vi "R45crio2_fpga.vi"() -> ()   [LabVIEW 2016]
uses:
  <vilib>/LabVIEW Targets/FPGA/cRIO/shared/nicrio_ModuleControls/nicrio_cRIO-9871_BaudRateEnum.ctl
  <vilib>/LabVIEW Targets/FPGA/cRIO/shared/nicrio_ModuleControls/nicrio_cRIO-9871_DataBitsEnum.ctl
  <vilib>/LabVIEW Targets/FPGA/cRIO/shared/nicrio_ModuleControls/nicrio_cRIO-9871_StopBitsEnum.ctl
  <vilib>/LabVIEW Targets/FPGA/cRIO/shared/nicrio_ModuleControls/nicrio_cRIO-9871_ParityEnum.ctl
  <vilib>/Platform/TimedLoop/XDataNode/timing_clust.ctl
  <vilib>/Platform/TimedLoop/XDataNode/nitl_modes.ctl
  <vilib>/Platform/TimedLoop/XDataNode/wakeup.ctl
  <vilib>/rvi/FXPMathLib/basic elements/FxpIntAccumulator/subVIs/nifxpmath_IntAccumulator_SimConfig.ctl
  <vilib>/rvi/Emulation/niFpgaGetClockAttributes.vi
  <vilib>/rvi/Emulation/niFpgaSctlEmulationGetInTimedLoop.vi
  <vilib>/rvi/Emulation/niFpgaEmulationReportErrorSimple.vi
  <vilib>/rvi/eio/common/nirviEmuTemplateMethod_errors.vi
  <vilib>/rvi/Emulation/niFpgaCriticalErrorInLSC.vi
  <vilib>/rvi/Analysis/common/codeGenErrors/XNode/niFpgaXNodeCodeGenErrorHandle.vi
  <vilib>/rvi/FXPMathLib/basic elements/FxpIntAccumulator/simVIs/DllFxpIntAccumulator_sub.vi
  <vilib>/rvi/eio/common/nirviEmuTemplatePropertySet_noerrors.vi
  <vilib>/eio/EIONode/EIONode.xnode
  <vilib>/eio/EIOMethodNode/EIOMethodNode.xnode
  <vilib>/rvi/Analysis/measure/dc-rms/XNode/niFpgaDC-RMS.xnode
  <vilib>/Platform/TimedLoop/XDataNode/XDataNode.xnode
  <vilib>/rvi/FXPMathLib/basic elements/FxpIntAccumulator/XNode/nifxpmath_IntAccumulator.xnode
  <vilib>/rvi/FXPMathLib/FxpMul/XNode/nifxpmath_Multiplier.xnode
  <vilib>/eio/EIOPropertyNode/EIOPropertyNode.xnode
  <vilib>/Platform/TimedLoop/XDataNode/XDNodeRunTimeDep.lvlib
  <vilib>/rvi/FXPMathLib/sim/FxpSim.dll
  <vilib>/rvi/eio/common/nirviEmuTemplatePropertyGet_errors.vi
  <vilib>/rvi/eio/common/nirviEmuTemplatePropertyGet_noerrors.vi
  <vilib>/rvi/eio/common/nirviEmuTemplatePropertySet_errors.vi
panel:
  out "ig":bool
  out "cg gauge":bool
  in  "turbo valve R45 ExB":bool
  in  "beamline valve R45 detector":bool
  in  "turbo valve r45 det turbo":bool
  in  "turbo valve r45 waist":bool
  out "Data":u8
  out "Timed Out":bool
  out "gfm read":u8[](array[numeric])
  in  "gfm set field array":u8[](array[numeric])=[0, 0, 0, 0, 0, 0, 0, 0, 0, 0]
  out "Reset 2":bool
  in  "Reset":bool
  in  "exb ps set array 2":u8[](array[numeric])=[0, 0, 0, 0, 0, 0, 0, 0, 0, 0]
  out "r45 #4 Ion gauge 2":u8[](array[numeric])
  out "r45 #4 Convectron 2":u8[](array[numeric])
  out "r45 #4 Convectron 1":u8[](array[numeric])
  out "r45 #4 Ion gauge 1":u8[](array[numeric])
  out "r45 #3 Ion gauge 2":u8[](array[numeric])
  out "r45 #3 Convectron 2":u8[](array[numeric])
  out "r45 #3 Convectron 1":u8[](array[numeric])
  out "r45 #3 Ion gauge 1":u8[](array[numeric])
  out "r45 #2 Ion gauge 2":u8[](array[numeric])
  out "r45 #2 Convectron 2":u8[](array[numeric])
  out "r45 #2 Convectron 1":u8[](array[numeric])
  out "r45 #2 Ion gauge 1":u8[](array[numeric])
  in  "exb ps set array":u8[](array[numeric])=[0, 0, 0, 0, 0, 0, 0, 0, 0, 0]
  out "DIO OUTPUT":bool[](array[boolean])
  in  "R45 det  faraday cup":bool
  in  "R45 det Aperture":bool
  out "Analog input":fxp<+/-,26,5>[](array[numeric]) format="%.23g"
  in  "Analog Output":fxp<+/-,26,5>[](array[numeric])=[0.0, 0.0, 0.0, 0.0, 0.0, 0.0, 0.0, 0.0] format="%.23g"
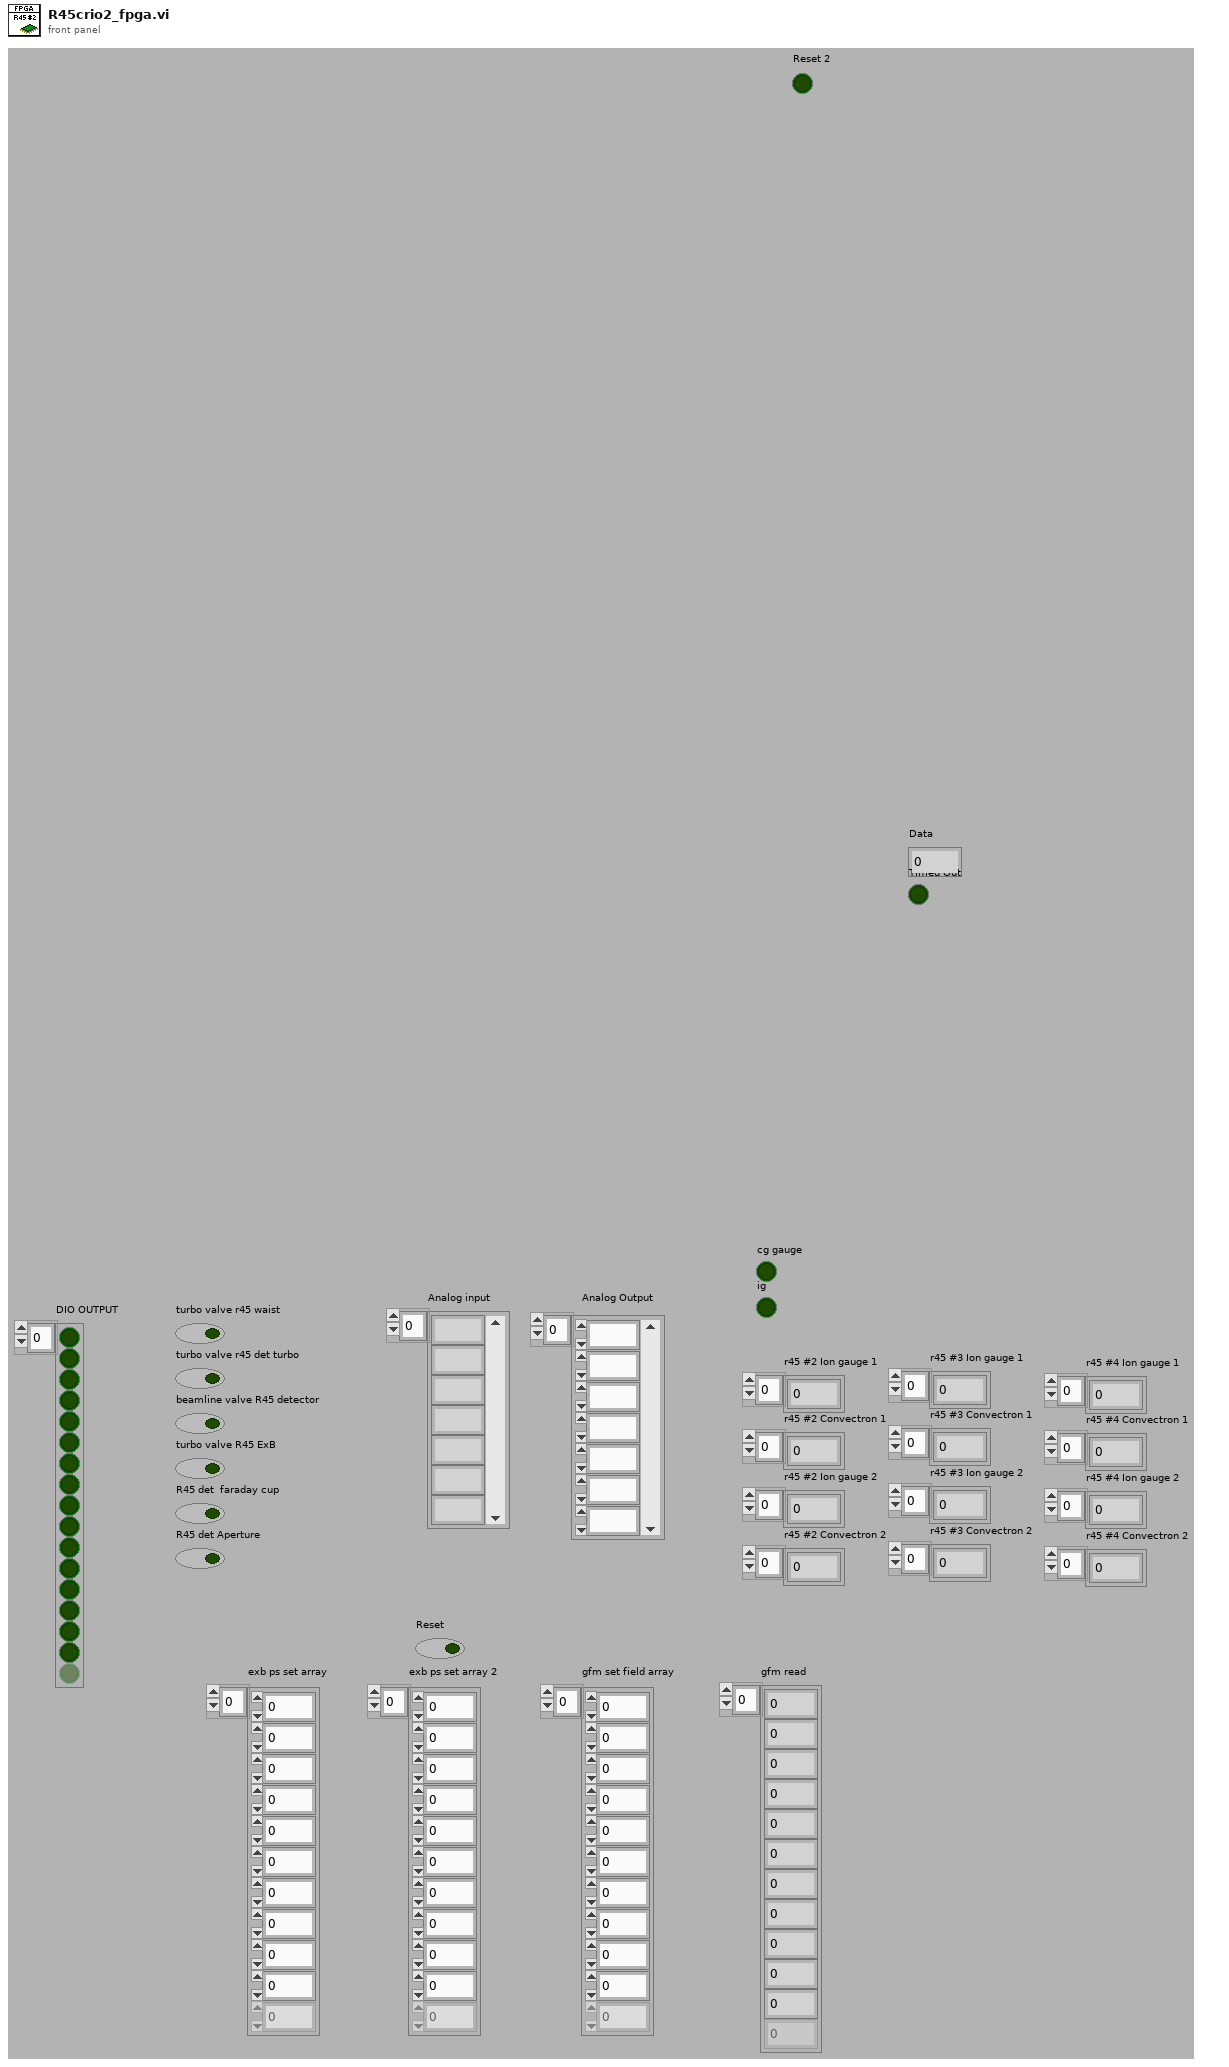
[diagram p1: front panel]
types:
  T1 = typedef "nicrio_cRIO-9871_ParityEnum.ctl" = enum8{"None", "Odd", "Even", "Mark", "Space"}
  T2 = typedef "nicrio_cRIO-9871_StopBitsEnum.ctl" = enum8{"1", "1.5", "2"}
  T3 = typedef "nicrio_cRIO-9871_BaudRateEnum.ctl" = enum16{"75 bps", "110 bps", "134 bps", "150 bps", "300 bps", "600 bps", "1200 bps", "1800 bps", "2400 bps", "4800 bps", "7200 bps", "9600 bps", "14.4 kbps", "19.2 kbps", "28.8 kbps", "38.4 kbps", "57.6 kbps", "115.2 kbps", "230.4 kbps", "460.8 kbps", "921.6 kbps"}
  T4 = typedef "nicrio_cRIO-9871_DataBitsEnum.ctl" = enum8{"5", "6", "7", "8"}
  T5 = typedef "XDNodeRunTimeDep.lvlib/timing_clust.ctl" = cluster{"Expected End [f-1]":u64, "Actual End [f-1]":u64, "Finished Late? [f-1]":bool, "Expected End [i-1]":u64, "Actual End [i-1]":u64, "Finished Late? [i-1]":bool, "Expected Start [i]":u64, "Actual Start [i]":u64, "Expected Start [f]":u64, "Actual Start [f]":u64, "Source Name":string, "Structure Name":string, "Period":i64, "Deadline":i64, "Offset":i64, "Start":i64, "Priority":i32, "Timeout":i32, "Mode":T6, "Wakeup Reason":T7, "Error":errorcluster, "Source Type":string, "Secondary Source Type":string, "Global End Time":u64, "Global Start Time":u64, "Frame Duration":u64, "Iteration Duration":u64, "Assigned CPU":i32, "I/O Scan Engine Mode":u32}
  T6 = typedef "XDNodeRunTimeDep.lvlib/nitl_modes.ctl" = enum32{"No Change", "Process missed periods, maintain original phase", "Discard missed periods, maintain original phase", "Process missed periods, ignore original phase", "Discard missed periods, ignore original phase"}
  T7 = typedef "XDNodeRunTimeDep.lvlib/wakeup.ctl" = enum32{"Normal", "Aborted", "Asynchronous wakeup", "Timing source error", "Timed loop error", "Timeout"}
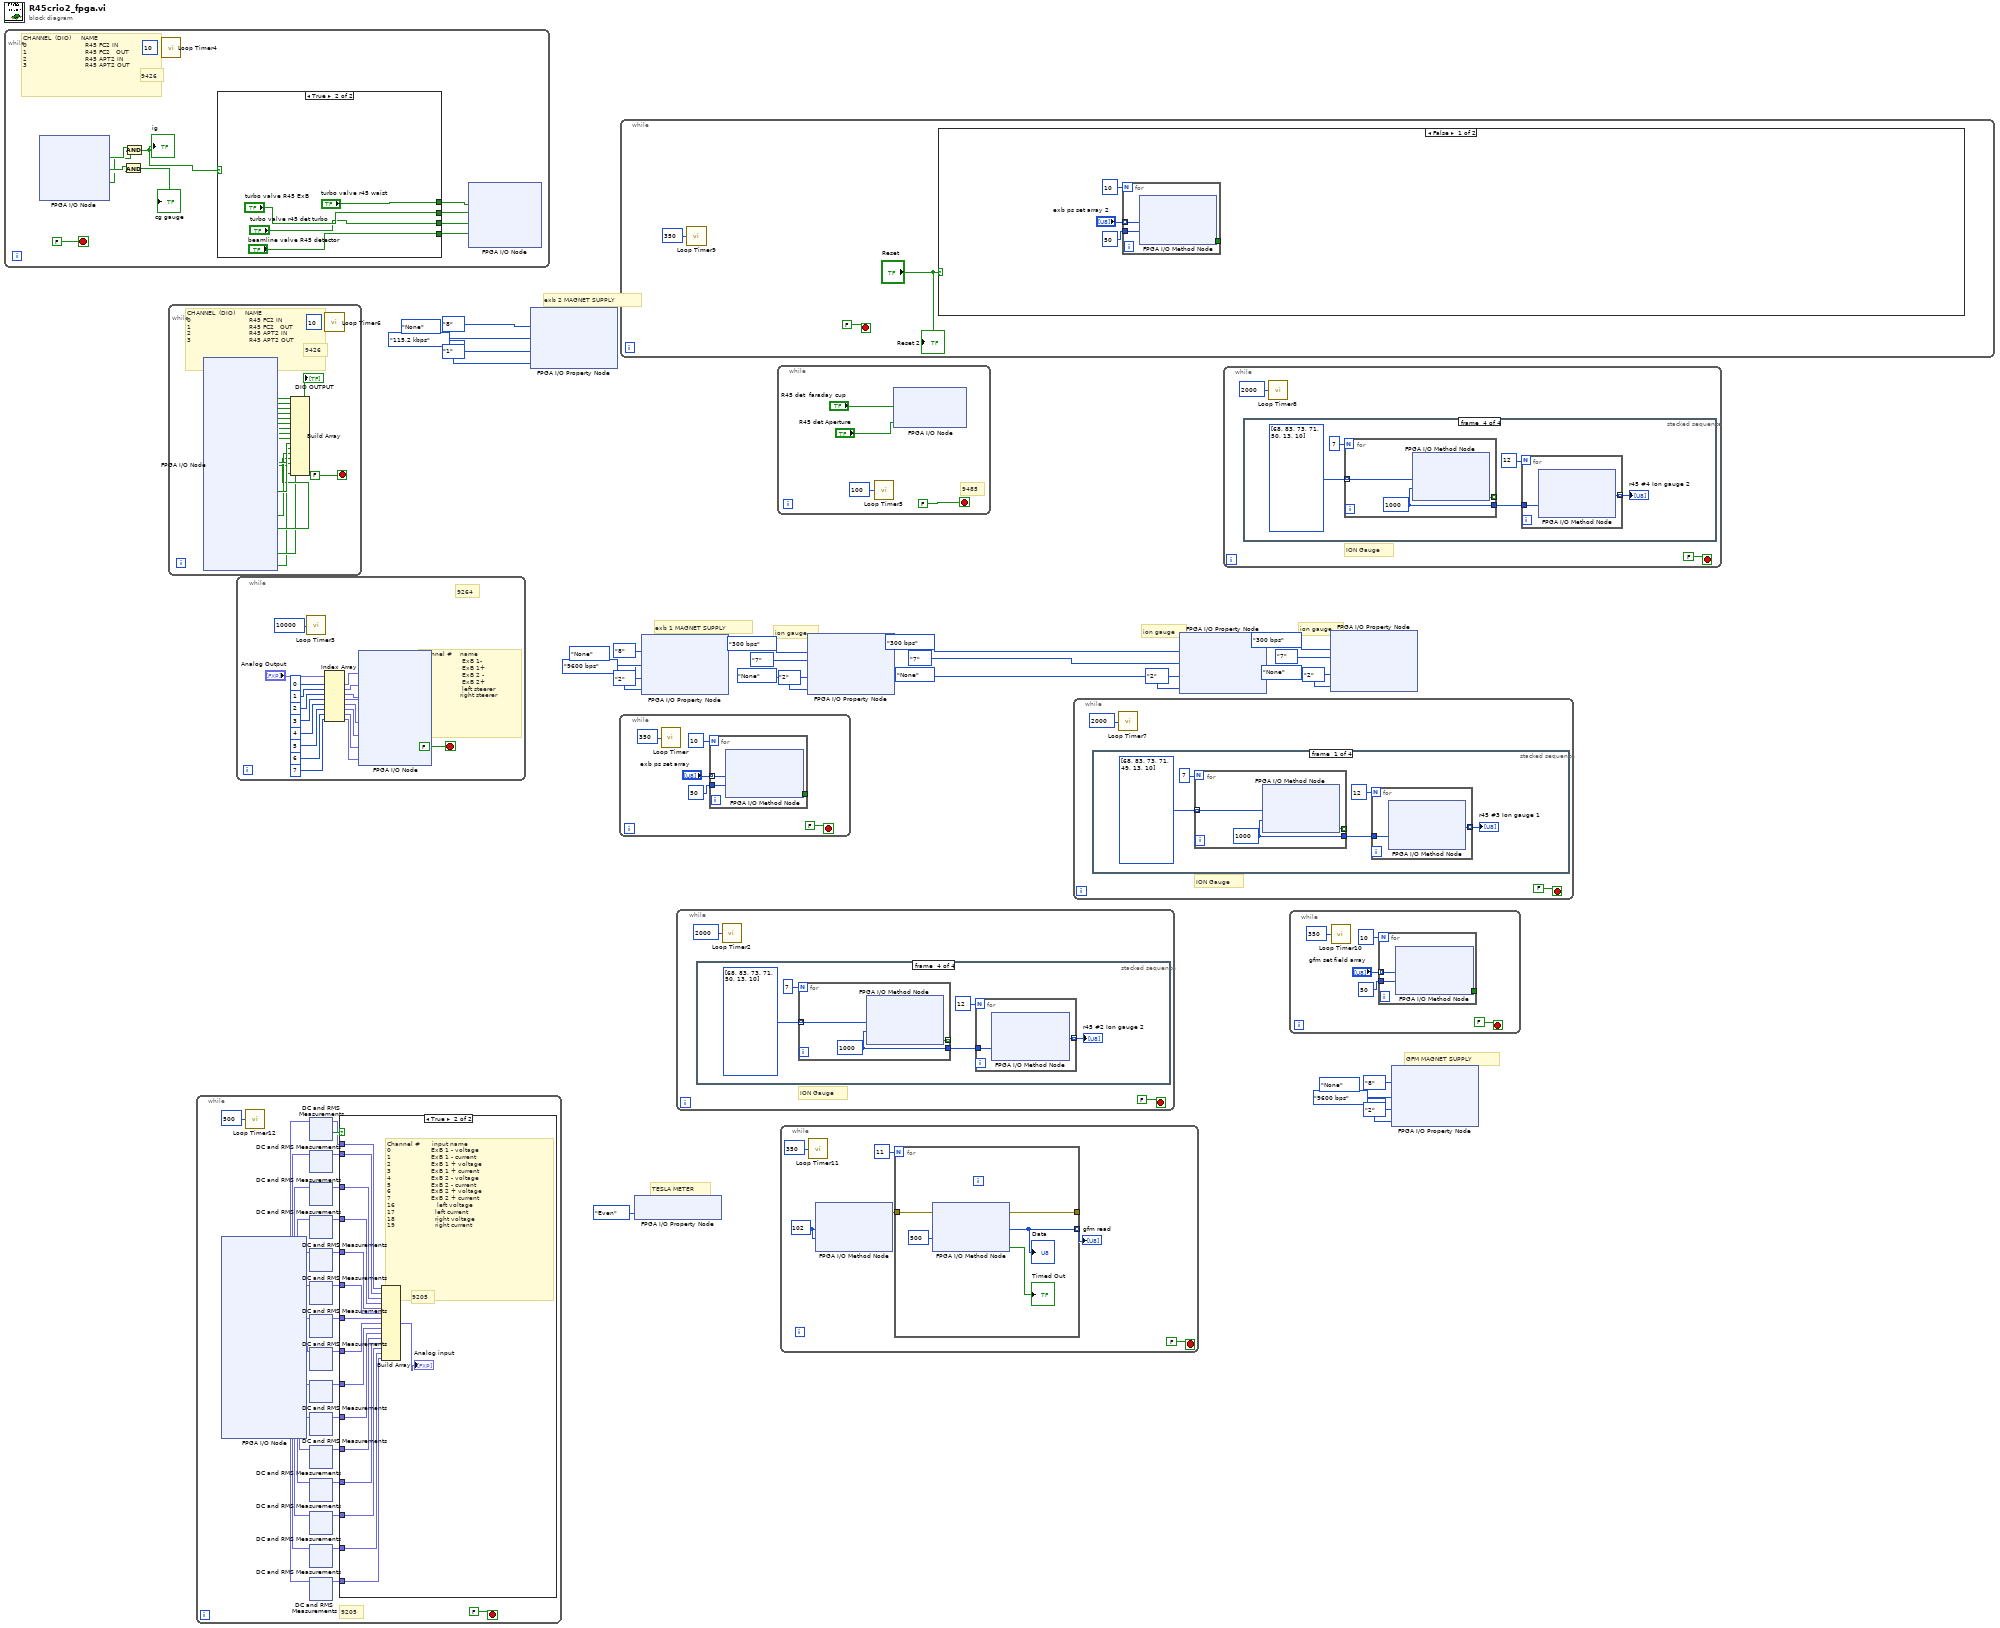
[diagram p0: block diagram]
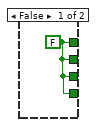
[diagram p2: hidden frame]
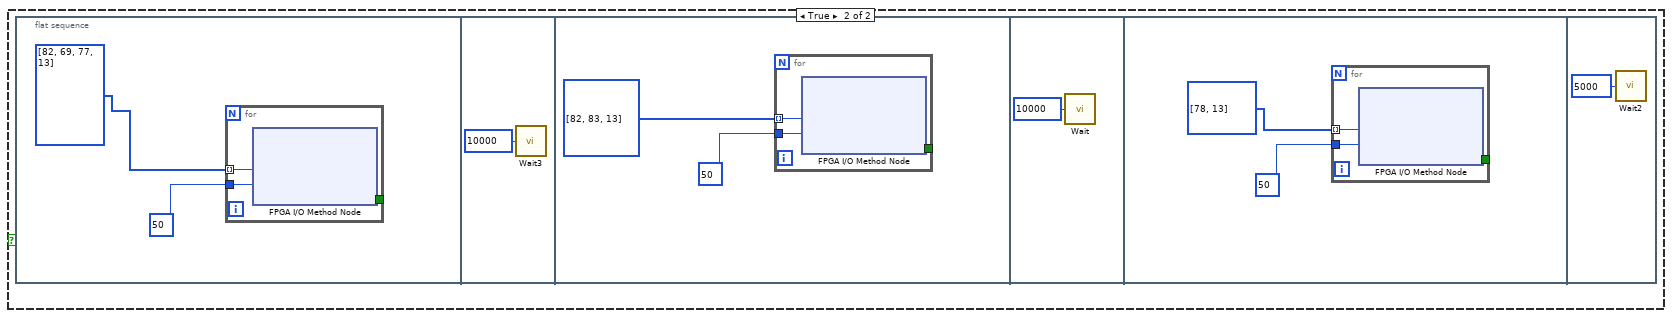
[diagram p4: hidden frame]
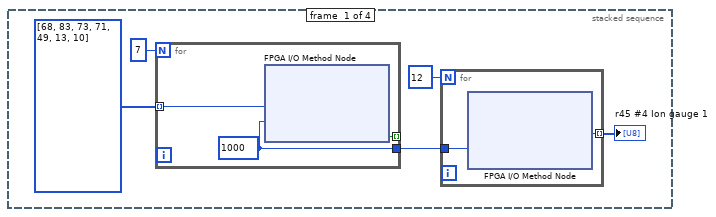
[diagram p5: hidden frame]
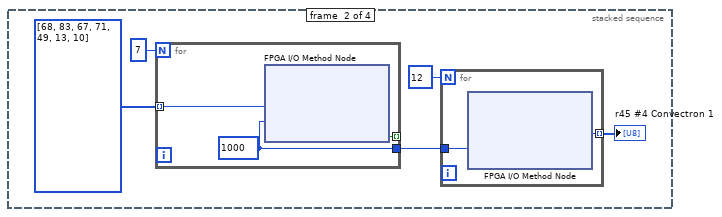
[diagram p6: hidden frame]
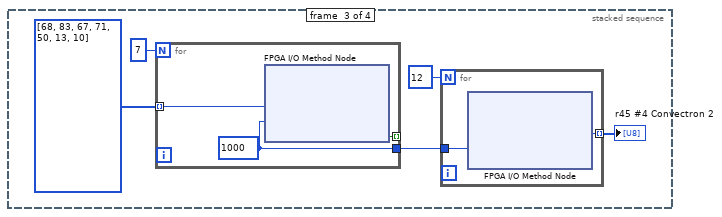
[diagram p7: hidden frame]
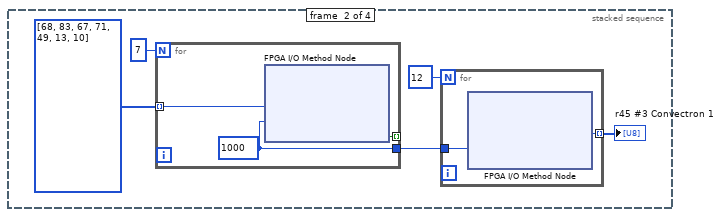
[diagram p8: hidden frame]
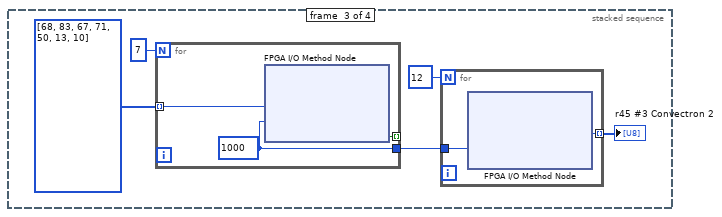
[diagram p9: hidden frame]
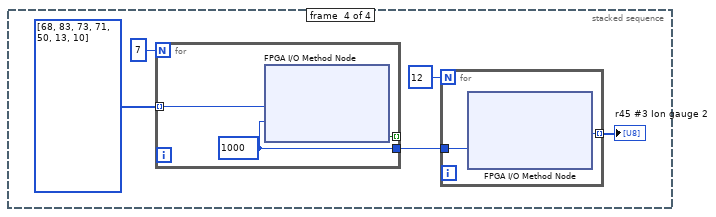
[diagram p10: hidden frame]
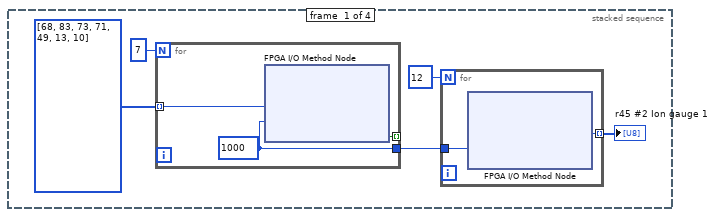
[diagram p11: hidden frame]
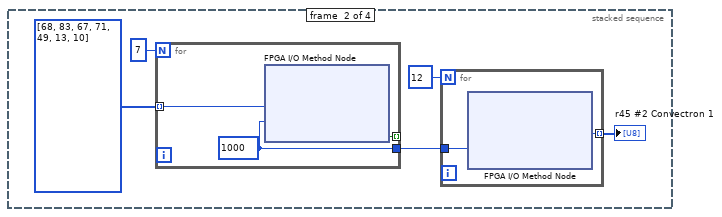
[diagram p12: hidden frame]
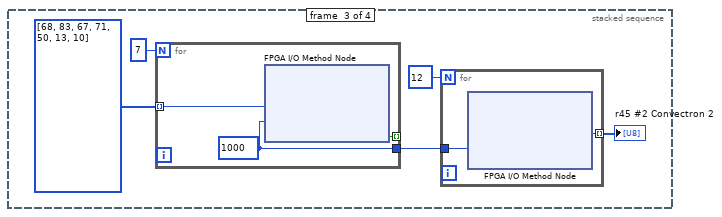
[diagram p13: hidden frame]
diagram:
  # "TESLA METER"
  # "GFM MAGNET SUPPLY"
  # "exb 2 MAGNET SUPPLY"
  # "ion gauge"
  # "ion gauge"
  # "ion gauge"
  # "exb 1 MAGNET SUPPLY"
  n1 = while {
    stop <- FALSE stop-if-true
    # "9426"
    # "CHANNEL  (DIO)     NAME\n0                             R45 FC2 IN\n1                             R45 FC2   OUT\n2                             R45 APT2 IN\n3                             R45 APT2 OUT"
    n2 = xnode "FPGA I/O Node"() -> ("Mod7/DI5"=w28:bool, "Mod7/DI6"=w35:bool, "Mod7/DI7"=w27:bool, "Mod7/DI8"=w34:bool)  [unwired: 4 in, 4 out]
    n3 = And(x=w35, y=w34) -> (x .and. y?=→"cg gauge":bool)
    n4 = And(x=w28, y=w27) -> (x .and. y?=w26:bool)
    "ig" <- w26
    n5 = call "Loop Timer4"("Count(uSec)"=u32 10 ("Count(Ticks)")) -> ()  [unwired: 1 out]
    n6 = case shown="True" w26 {
      tunnel: [w38 "turbo valve r45 waist"] -> w33
      tunnel: [w38 "turbo valve R45 ExB"] -> w32
      tunnel: [w38 "turbo valve r45 det turbo"] -> w31
      tunnel: [w38 "beamline valve R45 detector"] -> w30
      frame False {
        w38 = FALSE ("turbo valve r45 waist")
      }
      frame True {
      }
    }
    n7 = xnode "FPGA I/O Node"("Mod8/CH3"=w33, "Mod8/CH4"=w32, "Mod8/CH5"=w31, "Mod8/CH6"=w30) -> ()  [unwired: 4 in, 4 out]
  }
  n8 = while {
    stop <- FALSE stop-if-true
    # "9426"
    # "CHANNEL  (DIO)     NAME\n0                             R45 FC2 IN\n1                             R45 FC2   OUT\n2                             R45 APT2 IN\n3                             R45 APT2 OUT"
    n9 = xnode "FPGA I/O Node"() -> ("Mod7/DI0"=w55:bool, "Mod7/DI1"=w56:bool, "Mod7/DI2"=w57:bool, "Mod7/DI3"=w58:bool, "Mod7/DI4"=w54:bool, "Mod7/DI5"=w53:bool, "Mod7/DI6"=w52:bool, "Mod7/DI7"=w51:bool, "Mod7/DI8"=w50:bool, "Mod7/DI9"=w49:bool, "Mod7/DI10"=w48:bool, "Mod7/DI11"=w47:bool, "Mod7/DI12"=w46:bool, "Mod7/DI13"=w45:bool, "Mod7/DI14"=w44:bool, "Mod7/DI15"=w43:bool)  [unwired: 16 in, 16 out]
    n10 = Build Array(w55, w56, w57, w58, w54, w53, w52, w51, w50, w49, w48, w47, w46, w45, w44, w43) -> (→"DIO OUTPUT":bool[])
    n11 = call "Loop Timer6"("Count(uSec)"=u32 10 ("Count(Ticks)")) -> ()  [unwired: 1 out]
  }
  n12 = while {
    stop <- FALSE stop-if-true
    # "9205"
    n13 = xnode "FPGA I/O Node"() -> ("ExB 1- V read"=w91:fxp<+/-,26,5>, "ExB 1- I read"=w89:fxp<+/-,26,5>, "ExB 1+ V read"=w87:fxp<+/-,26,5>, "ExB 1+ I read"=w85:fxp<+/-,26,5>, "ExB 2- V read"=w83:fxp<+/-,26,5>, "ExB 2- I read"=w81:fxp<+/-,26,5>, "ExB 2+ V read"=w79:fxp<+/-,26,5>, "ExB 2+ I read"=w77:fxp<+/-,26,5>, "Mod1/AI16"=w75:fxp<+/-,26,5>, "Mod1/AI17"=w73:fxp<+/-,26,5>, "Mod1/AI18"=w71:fxp<+/-,26,5>, "Mod1/AI19"=w69:fxp<+/-,26,5>, "Mod1/AI20"=w67:fxp<+/-,26,5>, "Mod1/AI21"=w65:fxp<+/-,26,5>, "Mod1/AI22"=w63:fxp<+/-,26,5>)  [unwired: 15 in, 15 out]
    n14 = call "Loop Timer12"("Count(Ticks)"=u32 500) -> ()  [unwired: 1 out]
    n15 = xnode "DC and RMS Measurements"("input data"=w91) -> ("DC"=w90:fxp<+/-,26,5>, "output valid"=w92:bool)  [unwired: 1 in]
    n16 = xnode "DC and RMS Measurements"("input data"=w89) -> ("DC"=w88:fxp<+/-,26,5>)  [unwired: 1 in, 1 out]
    n17 = xnode "DC and RMS Measurements"("input data"=w87) -> ("DC"=w86:fxp<+/-,26,5>)  [unwired: 1 in, 1 out]
    n18 = xnode "DC and RMS Measurements"("input data"=w85) -> ("DC"=w84:fxp<+/-,26,5>)  [unwired: 1 in, 1 out]
    n19 = xnode "DC and RMS Measurements"("input data"=w83) -> ("DC"=w82:fxp<+/-,26,5>)  [unwired: 1 in, 1 out]
    n20 = xnode "DC and RMS Measurements"("input data"=w81) -> ("DC"=w80:fxp<+/-,26,5>)  [unwired: 1 in, 1 out]
    n21 = xnode "DC and RMS Measurements"("input data"=w79) -> ("DC"=w78:fxp<+/-,26,5>)  [unwired: 1 in, 1 out]
    n22 = xnode "DC and RMS Measurements"("input data"=w77) -> ("DC"=w76:fxp<+/-,26,5>)  [unwired: 1 in, 1 out]
    n23 = xnode "DC and RMS Measurements"("input data"=w75) -> ("DC"=w74:fxp<+/-,26,5>)  [unwired: 1 in, 1 out]
    n24 = xnode "DC and RMS Measurements"("input data"=w73) -> ("DC"=w72:fxp<+/-,26,5>)  [unwired: 1 in, 1 out]
    n25 = xnode "DC and RMS Measurements"("input data"=w71) -> ("DC"=w70:fxp<+/-,26,5>)  [unwired: 1 in, 1 out]
    n26 = xnode "DC and RMS Measurements"("input data"=w69) -> ("DC"=w68:fxp<+/-,26,5>)  [unwired: 1 in, 1 out]
    n27 = xnode "DC and RMS Measurements"("input data"=w67) -> ("DC"=w66:fxp<+/-,26,5>)  [unwired: 1 in, 1 out]
    n28 = xnode "DC and RMS Measurements"("input data"=w65) -> ("DC"=w64:fxp<+/-,26,5>)  [unwired: 1 in, 1 out]
    n29 = xnode "DC and RMS Measurements"("input data"=w63) -> ("DC"=w62:fxp<+/-,26,5>)  [unwired: 1 in, 1 out]
    n30 = case shown="True" w92 {
      tunnel: w90 -> [_ w270]
      tunnel: w88 -> [_ w269]
      tunnel: w86 -> [_ w268]
      tunnel: w84 -> [_ w267]
      tunnel: w82 -> [_ w266]
      tunnel: w80 -> [_ w265]
      tunnel: w78 -> [_ w264]
      tunnel: w76 -> [_ w263]
      tunnel: w74 -> [_ w262]
      tunnel: w72 -> [_ w261]
      tunnel: w70 -> [_ w260]
      tunnel: w68 -> [_ w259]
      tunnel: w66 -> [_ w258]
      tunnel: w64 -> [_ w257]
      tunnel: w62 -> [_ w256]
      frame False {
      }
      frame True {
        # "Channel #      input name\n0                    ExB 1 - voltage\n1                    ExB 1 - current\n2                    ExB 1 + voltage\n3                    ExB 1 + current\n4                    ExB 2 - voltage\n5                    ExB 2 - current\n6                    ExB 2 + voltage\n7                    ExB 2 + current                   \n16                     left voltage\n17                    left current\n18                    right voltage\n19                    right current"
        # "9205"
        n31 = Build Array(w270, w269, w268, w267, w266, w265, w264, w263, w262, w261, w260, w259, w258, w257, w256) -> (→"Analog input":fxp<+/-,26,5>[])
      }
    }
  }
  n32 = while {
    stop <- FALSE stop-if-true
    # "channel #    name\n0                   ExB 1-\n1                   ExB 1+\n2                   ExB 2 -\n3                   ExB 2+\n4                   left steerer\n5                  right steerer"
    # "9264"
    n33 = call "Loop Timer3"("Count(Ticks)"=u32 10000) -> ()  [unwired: 1 out]
    n34 = Index Array(array="Analog Output", index #1=0 ("index"), index #2=1 ("index"), index #3=2 ("index"), index #4=3 ("index"), index #5=4 ("index"), index #6=5 ("index"), index #7=6 ("index"), index #8=7 ("index")) -> (element #1=w1322:fxp<+/-,26,5>, element #2=w1321:fxp<+/-,26,5>, element #3=w1320:fxp<+/-,26,5>, element #4=w1319:fxp<+/-,26,5>, element #5=w1314:fxp<+/-,26,5>, element #6=w1313:fxp<+/-,26,5>, element #7=w1312:fxp<+/-,26,5>, element #8=w1311:fxp<+/-,26,5>)
    n35 = xnode "FPGA I/O Node"("Mod2/AO0"=w1322, "Mod2/AO1"=w1321, "Mod2/AO2"=w1320, "Mod2/AO3"=w1319, "Mod2/AO4"=w1314, "Mod2/AO5"=w1313, "Mod2/AO6"=w1312, "Mod2/AO7"=w1311) -> ()  [unwired: 8 in, 8 out]
  }
  n36 = xnode "FPGA I/O Property Node"("Data Bits"=nicrio_cRIO-9871_DataBitsEnum."8", "Parity"=nicrio_cRIO-9871_ParityEnum."None", "Baud Rate"=nicrio_cRIO-9871_BaudRateEnum."115.2 kbps", "Stop Bits"=nicrio_cRIO-9871_StopBitsEnum."1") -> ()  [unwired: 1 in, 1 out]
  n37 = while {
    stop <- FALSE stop-if-true
    n38 = call "Loop Timer"("Count(mSec)"=u32 350) -> ()  [unwired: 1 out]
    n39 = for {
      N: 10 -> [_]
      tunnel: 50 ("Timeout (ms)") -> [w1337]
      tunnel: "exb ps set array" -> [w1336] mode=indexing
      tunnel: [w1335] -> _
      n40 = xnode "FPGA I/O Method Node"("Data"=w1336, "Timeout (ms)"=w1337) -> ("Timed Out"=w1335:bool)  [unwired: 2 in, 2 out]
    }
  }
  n41 = while {
    stop <- FALSE stop-if-true
    n42 = call "Loop Timer9"("Count(mSec)"=u32 350) -> ()  [unwired: 1 out]
    n43 = case shown="False" "Reset" {
      frame False {
        n44 = for {
          N: 10 -> [_]
          tunnel: 50 ("Timeout (ms)") -> [w1346]
          tunnel: "exb ps set array 2" -> [w1345] mode=indexing
          tunnel: [w1344] -> _
          n45 = xnode "FPGA I/O Method Node"("Data"=w1345, "Timeout (ms)"=w1346) -> ("Timed Out"=w1344:bool)  [unwired: 2 in, 2 out]
        }
      }
      frame True {
        n46 = flat-sequence {
          frame #0 {
            n47 = for {
              tunnel: 50 ("Timeout (ms)") -> [w1351]
              tunnel: u8[] [82, 69, 77, 13] ("unsigned byte array") -> [w1350] mode=indexing
              tunnel: [w1349] -> _
              n48 = xnode "FPGA I/O Method Node"("Data"=w1350, "Timeout (ms)"=w1351) -> ("Timed Out"=w1349:bool)  [unwired: 2 in, 2 out]
            }
          }
          frame #1 {
            n49 = call "Wait3"("Count(mSec)"=u32 10000) -> ()  [unwired: 1 out]
          }
          frame #2 {
            n50 = for {
              tunnel: 50 ("Timeout (ms)") -> [w1357]
              tunnel: u8[] [82, 83, 13] ("unsigned byte array") -> [w1356] mode=indexing
              tunnel: [w1355] -> _
              n51 = xnode "FPGA I/O Method Node"("Data"=w1356, "Timeout (ms)"=w1357) -> ("Timed Out"=w1355:bool)  [unwired: 2 in, 2 out]
            }
          }
          frame #3 {
            n52 = call "Wait"("Count(mSec)"=u32 10000) -> ()  [unwired: 1 out]
          }
          frame #4 {
            n53 = for {
              tunnel: 50 ("Timeout (ms)") -> [w1363]
              tunnel: u8[] [78, 13] ("unsigned byte array") -> [w1362] mode=indexing
              tunnel: [w1361] -> _
              n54 = xnode "FPGA I/O Method Node"("Data"=w1362, "Timeout (ms)"=w1363) -> ("Timed Out"=w1361:bool)  [unwired: 2 in, 2 out]
            }
          }
          frame #5 {
            n55 = call "Wait2"("Count(mSec)"=u32 5000) -> ()  [unwired: 1 out]
          }
        }
      }
    }
    "Reset 2" <- "Reset"
  }
  n56 = xnode "FPGA I/O Property Node"("Parity"=nicrio_cRIO-9871_ParityEnum."Even") -> ()  [unwired: 1 in, 1 out]
  n57 = xnode "FPGA I/O Property Node"("Data Bits"=nicrio_cRIO-9871_DataBitsEnum."8", "Parity"=nicrio_cRIO-9871_ParityEnum."None", "Baud Rate"=nicrio_cRIO-9871_BaudRateEnum."9600 bps", "Stop Bits"=nicrio_cRIO-9871_StopBitsEnum."2") -> ()  [unwired: 1 in, 1 out]
  n58 = while {
    stop <- FALSE stop-if-true
    # "ION Gauge"
    n59 = stacked-sequence {
      frame #0 {
        n60 = for {
          N: 7 -> [_]
          tunnel: [w1376] -> w1371
          tunnel: [w1375] -> _ mode=indexing
          tunnel: u8[] [68, 83, 73, 71, 49, 13, 10] ("unsigned byte array") -> [w1374] mode=indexing
          w1376 = 1000 ("Timeout (ms)")
          n61 = xnode "FPGA I/O Method Node"("Data"=w1374, "Timeout (ms)"=w1376) -> ("Timed Out"=w1375:bool)  [unwired: 1 in, 1 out]
        }
        n62 = for {
          N: 12 -> [_]
          tunnel: w1371 -> [w1373]
          tunnel: [w1372] -> w1367 mode=indexing
          n63 = xnode "FPGA I/O Method Node"("Timeout (ms)"=w1373) -> ("Data"=w1372:u8)  [unwired: 1 in, 2 out]
        }
        "r45 #2 Ion gauge 1" <- w1367
      }
      frame #1 {
        n64 = for {
          N: 7 -> [_]
          tunnel: [w1386] -> w1381
          tunnel: [w1385] -> _ mode=indexing
          tunnel: u8[] [68, 83, 67, 71, 49, 13, 10] ("unsigned byte array") -> [w1384] mode=indexing
          w1386 = 1000 ("Timeout (ms)")
          n65 = xnode "FPGA I/O Method Node"("Data"=w1384, "Timeout (ms)"=w1386) -> ("Timed Out"=w1385:bool)  [unwired: 1 in, 1 out]
        }
        n66 = for {
          N: 12 -> [_]
          tunnel: w1381 -> [w1383]
          tunnel: [w1382] -> w1377 mode=indexing
          n67 = xnode "FPGA I/O Method Node"("Timeout (ms)"=w1383) -> ("Data"=w1382:u8)  [unwired: 1 in, 2 out]
        }
        "r45 #2 Convectron 1" <- w1377
      }
      frame #2 {
        n68 = for {
          N: 7 -> [_]
          tunnel: [w1396] -> w1391
          tunnel: [w1395] -> _ mode=indexing
          tunnel: u8[] [68, 83, 67, 71, 50, 13, 10] ("unsigned byte array") -> [w1394] mode=indexing
          w1396 = 1000 ("Timeout (ms)")
          n69 = xnode "FPGA I/O Method Node"("Data"=w1394, "Timeout (ms)"=w1396) -> ("Timed Out"=w1395:bool)  [unwired: 1 in, 1 out]
        }
        n70 = for {
          N: 12 -> [_]
          tunnel: w1391 -> [w1393]
          tunnel: [w1392] -> w1387 mode=indexing
          n71 = xnode "FPGA I/O Method Node"("Timeout (ms)"=w1393) -> ("Data"=w1392:u8)  [unwired: 1 in, 2 out]
        }
        "r45 #2 Convectron 2" <- w1387
      }
      frame #3 {
        n72 = for {
          N: 7 -> [_]
          tunnel: [w1406] -> w1401
          tunnel: [w1405] -> _ mode=indexing
          tunnel: u8[] [68, 83, 73, 71, 50, 13, 10] ("unsigned byte array") -> [w1404] mode=indexing
          w1406 = 1000 ("Timeout (ms)")
          n73 = xnode "FPGA I/O Method Node"("Data"=w1404, "Timeout (ms)"=w1406) -> ("Timed Out"=w1405:bool)  [unwired: 1 in, 1 out]
        }
        n74 = for {
          N: 12 -> [_]
          tunnel: w1401 -> [w1403]
          tunnel: [w1402] -> w1397 mode=indexing
          n75 = xnode "FPGA I/O Method Node"("Timeout (ms)"=w1403) -> ("Data"=w1402:u8)  [unwired: 1 in, 2 out]
        }
        "r45 #2 Ion gauge 2" <- w1397
      }
    }
    n76 = call "Loop Timer2"("Count(mSec)"=u32 2000 ("Count(Ticks)")) -> ()  [unwired: 1 out]
  }
  n77 = while {
    stop <- FALSE stop-if-true
    # "9485"
    n78 = call "Loop Timer5"("Count(uSec)"=u32 100 ("Count(Ticks)")) -> ()  [unwired: 1 out]
    n79 = xnode "FPGA I/O Node"("Mod8/CH0"="R45 det  faraday cup", "Mod8/CH2"="R45 det Aperture") -> ()  [unwired: 2 in, 2 out]
  }
  n80 = while {
    stop <- FALSE stop-if-true
    w1413 = u8 102 ("Data")
    n81 = call "Loop Timer11"("Count(mSec)"=u32 350) -> ()  [unwired: 1 out]
    n82 = xnode "FPGA I/O Method Node"("Data"=w1413, "Timeout (ms)"=w1413) -> ("error out"=w1412:errorcluster)  [unwired: 2 in, 2 out]
    n83 = for {
      N: 11 ("Numeric 3") -> [_]
      tunnel: [w1419] -> w1414 mode=indexing
      tunnel: w1412 -> [w1418]
      tunnel: [w1417] -> _
      n84 = xnode "FPGA I/O Method Node"("error in"=w1418, "Timeout (ms)"=500) -> ("error out"=w1417:errorcluster, "Data"=w1419:u8, "Timed Out"=→"Timed Out":bool)  [unwired: 1 in, 1 out]
      "Data" <- w1419
    }
    "gfm read" <- w1414
  }
  n85 = xnode "FPGA I/O Property Node"("Baud Rate"=nicrio_cRIO-9871_BaudRateEnum."300 bps", "Data Bits"=nicrio_cRIO-9871_DataBitsEnum."7", "Parity"=nicrio_cRIO-9871_ParityEnum."None", "Stop Bits"=nicrio_cRIO-9871_StopBitsEnum."2") -> ()  [unwired: 1 in, 1 out]
  n86 = while {
    stop <- FALSE stop-if-true
    # "ION Gauge"
    n87 = stacked-sequence {
      frame #0 {
        n88 = for {
          N: 7 -> [_]
          tunnel: [w1433] -> w1428
          tunnel: [w1432] -> _ mode=indexing
          tunnel: u8[] [68, 83, 73, 71, 49, 13, 10] ("unsigned byte array") -> [w1431] mode=indexing
          w1433 = 1000 ("Timeout (ms)")
          n89 = xnode "FPGA I/O Method Node"("Data"=w1431, "Timeout (ms)"=w1433) -> ("Timed Out"=w1432:bool)  [unwired: 1 in, 1 out]
        }
        n90 = for {
          N: 12 -> [_]
          tunnel: w1428 -> [w1430]
          tunnel: [w1429] -> w1424 mode=indexing
          n91 = xnode "FPGA I/O Method Node"("Timeout (ms)"=w1430) -> ("Data"=w1429:u8)  [unwired: 1 in, 2 out]
        }
        "r45 #3 Ion gauge 1" <- w1424
      }
      frame #1 {
        n92 = for {
          N: 7 -> [_]
          tunnel: [w1443] -> w1438
          tunnel: [w1442] -> _ mode=indexing
          tunnel: u8[] [68, 83, 67, 71, 49, 13, 10] ("unsigned byte array") -> [w1441] mode=indexing
          w1443 = 1000 ("Timeout (ms)")
          n93 = xnode "FPGA I/O Method Node"("Data"=w1441, "Timeout (ms)"=w1443) -> ("Timed Out"=w1442:bool)  [unwired: 1 in, 1 out]
        }
        n94 = for {
          N: 12 -> [_]
          tunnel: w1438 -> [w1440]
          tunnel: [w1439] -> w1434 mode=indexing
          n95 = xnode "FPGA I/O Method Node"("Timeout (ms)"=w1440) -> ("Data"=w1439:u8)  [unwired: 1 in, 2 out]
        }
        "r45 #3 Convectron 1" <- w1434
      }
      frame #2 {
        n96 = for {
          N: 7 -> [_]
          tunnel: [w1453] -> w1448
          tunnel: [w1452] -> _ mode=indexing
          tunnel: u8[] [68, 83, 67, 71, 50, 13, 10] ("unsigned byte array") -> [w1451] mode=indexing
          w1453 = 1000 ("Timeout (ms)")
          n97 = xnode "FPGA I/O Method Node"("Data"=w1451, "Timeout (ms)"=w1453) -> ("Timed Out"=w1452:bool)  [unwired: 1 in, 1 out]
        }
        n98 = for {
          N: 12 -> [_]
          tunnel: w1448 -> [w1450]
          tunnel: [w1449] -> w1444 mode=indexing
          n99 = xnode "FPGA I/O Method Node"("Timeout (ms)"=w1450) -> ("Data"=w1449:u8)  [unwired: 1 in, 2 out]
        }
        "r45 #3 Convectron 2" <- w1444
      }
      frame #3 {
        n100 = for {
          N: 7 -> [_]
          tunnel: [w1463] -> w1458
          tunnel: [w1462] -> _ mode=indexing
          tunnel: u8[] [68, 83, 73, 71, 50, 13, 10] ("unsigned byte array") -> [w1461] mode=indexing
          w1463 = 1000 ("Timeout (ms)")
          n101 = xnode "FPGA I/O Method Node"("Data"=w1461, "Timeout (ms)"=w1463) -> ("Timed Out"=w1462:bool)  [unwired: 1 in, 1 out]
        }
        n102 = for {
          N: 12 -> [_]
          tunnel: w1458 -> [w1460]
          tunnel: [w1459] -> w1454 mode=indexing
          n103 = xnode "FPGA I/O Method Node"("Timeout (ms)"=w1460) -> ("Data"=w1459:u8)  [unwired: 1 in, 2 out]
        }
        "r45 #3 Ion gauge 2" <- w1454
      }
    }
    n104 = call "Loop Timer7"("Count(mSec)"=u32 2000 ("Count(Ticks)")) -> ()  [unwired: 1 out]
  }
  n105 = xnode "FPGA I/O Property Node"("Baud Rate"=nicrio_cRIO-9871_BaudRateEnum."300 bps", "Data Bits"=nicrio_cRIO-9871_DataBitsEnum."7", "Parity"=nicrio_cRIO-9871_ParityEnum."None", "Stop Bits"=nicrio_cRIO-9871_StopBitsEnum."2") -> ()  [unwired: 1 in, 1 out]
  n106 = while {
    stop <- FALSE stop-if-true
    # "ION Gauge"
    n107 = stacked-sequence {
      frame #0 {
        n108 = for {
          N: 7 -> [_]
          tunnel: [w1475] -> w1470
          tunnel: [w1474] -> _ mode=indexing
          tunnel: u8[] [68, 83, 73, 71, 49, 13, 10] ("unsigned byte array") -> [w1473] mode=indexing
          w1475 = 1000 ("Timeout (ms)")
          n109 = xnode "FPGA I/O Method Node"("Data"=w1473, "Timeout (ms)"=w1475) -> ("Timed Out"=w1474:bool)  [unwired: 1 in, 1 out]
        }
        n110 = for {
          N: 12 -> [_]
          tunnel: w1470 -> [w1472]
          tunnel: [w1471] -> w1466 mode=indexing
          n111 = xnode "FPGA I/O Method Node"("Timeout (ms)"=w1472) -> ("Data"=w1471:u8)  [unwired: 1 in, 2 out]
        }
        "r45 #4 Ion gauge 1" <- w1466
      }
      frame #1 {
        n112 = for {
          N: 7 -> [_]
          tunnel: [w1485] -> w1480
          tunnel: [w1484] -> _ mode=indexing
          tunnel: u8[] [68, 83, 67, 71, 49, 13, 10] ("unsigned byte array") -> [w1483] mode=indexing
          w1485 = 1000 ("Timeout (ms)")
          n113 = xnode "FPGA I/O Method Node"("Data"=w1483, "Timeout (ms)"=w1485) -> ("Timed Out"=w1484:bool)  [unwired: 1 in, 1 out]
        }
        n114 = for {
          N: 12 -> [_]
          tunnel: w1480 -> [w1482]
          tunnel: [w1481] -> w1476 mode=indexing
          n115 = xnode "FPGA I/O Method Node"("Timeout (ms)"=w1482) -> ("Data"=w1481:u8)  [unwired: 1 in, 2 out]
        }
        "r45 #4 Convectron 1" <- w1476
      }
      frame #2 {
        n116 = for {
          N: 7 -> [_]
          tunnel: [w1495] -> w1490
          tunnel: [w1494] -> _ mode=indexing
          tunnel: u8[] [68, 83, 67, 71, 50, 13, 10] ("unsigned byte array") -> [w1493] mode=indexing
          w1495 = 1000 ("Timeout (ms)")
          n117 = xnode "FPGA I/O Method Node"("Data"=w1493, "Timeout (ms)"=w1495) -> ("Timed Out"=w1494:bool)  [unwired: 1 in, 1 out]
        }
        n118 = for {
          N: 12 -> [_]
          tunnel: w1490 -> [w1492]
          tunnel: [w1491] -> w1486 mode=indexing
          n119 = xnode "FPGA I/O Method Node"("Timeout (ms)"=w1492) -> ("Data"=w1491:u8)  [unwired: 1 in, 2 out]
        }
        "r45 #4 Convectron 2" <- w1486
      }
      frame #3 {
        n120 = for {
          N: 7 -> [_]
          tunnel: [w1505] -> w1500
          tunnel: [w1504] -> _ mode=indexing
          tunnel: u8[] [68, 83, 73, 71, 50, 13, 10] ("unsigned byte array") -> [w1503] mode=indexing
          w1505 = 1000 ("Timeout (ms)")
          n121 = xnode "FPGA I/O Method Node"("Data"=w1503, "Timeout (ms)"=w1505) -> ("Timed Out"=w1504:bool)  [unwired: 1 in, 1 out]
        }
        n122 = for {
          N: 12 -> [_]
          tunnel: w1500 -> [w1502]
          tunnel: [w1501] -> w1496 mode=indexing
          n123 = xnode "FPGA I/O Method Node"("Timeout (ms)"=w1502) -> ("Data"=w1501:u8)  [unwired: 1 in, 2 out]
        }
        "r45 #4 Ion gauge 2" <- w1496
      }
    }
    n124 = call "Loop Timer8"("Count(mSec)"=u32 2000 ("Count(Ticks)")) -> ()  [unwired: 1 out]
  }
  n125 = while {
    stop <- FALSE stop-if-true
    n126 = call "Loop Timer10"("Count(mSec)"=u32 350) -> ()  [unwired: 1 out]
    n127 = for {
      N: 10 -> [_]
      tunnel: 50 ("Timeout (ms)") -> [w1513]
      tunnel: "gfm set field array" -> [w1512] mode=indexing
      tunnel: [w1511] -> _
      n128 = xnode "FPGA I/O Method Node"("Data"=w1512, "Timeout (ms)"=w1513) -> ("Timed Out"=w1511:bool)  [unwired: 2 in, 2 out]
    }
  }
  n129 = xnode "FPGA I/O Property Node"("Baud Rate"=nicrio_cRIO-9871_BaudRateEnum."300 bps", "Data Bits"=nicrio_cRIO-9871_DataBitsEnum."7", "Parity"=nicrio_cRIO-9871_ParityEnum."None", "Stop Bits"=nicrio_cRIO-9871_StopBitsEnum."2") -> ()  [unwired: 1 in, 1 out]
  n130 = xnode "FPGA I/O Property Node"("Data Bits"=nicrio_cRIO-9871_DataBitsEnum."8", "Parity"=nicrio_cRIO-9871_ParityEnum."None", "Baud Rate"=nicrio_cRIO-9871_BaudRateEnum."9600 bps", "Stop Bits"=nicrio_cRIO-9871_StopBitsEnum."2") -> ()  [unwired: 1 in, 1 out]
